vi "multiColorWormSaveSettings.vi"(1 "piezoPosition":dbl[](array[numeric]), 2 "moleculesSequence":string[](array[string])) -> ()   [LabVIEW 2017]
uses:
  globalUtilities.vi
  <vilib>/Utility/file.llb/Write Delimited Spreadsheet (DBL).vi
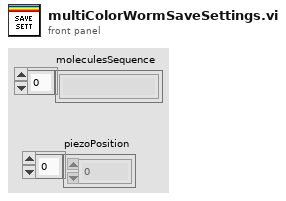
[diagram p1: front panel]
types:
  T1 = enum16{"open", "replace", "create", "open or create", "replace or create", "replace or create with confirmation"}
  T2 = cluster{"laserWavelength (nm)":dbl, "laserPower (mW)":dbl, "sliderPosition":u16}[]
  T3 = cluster{"laserWavelength":dbl, "exposureTime":dbl, "filterWheelPosition":u8, "name":string, "exposureTimeMultiplier":dbl}[]
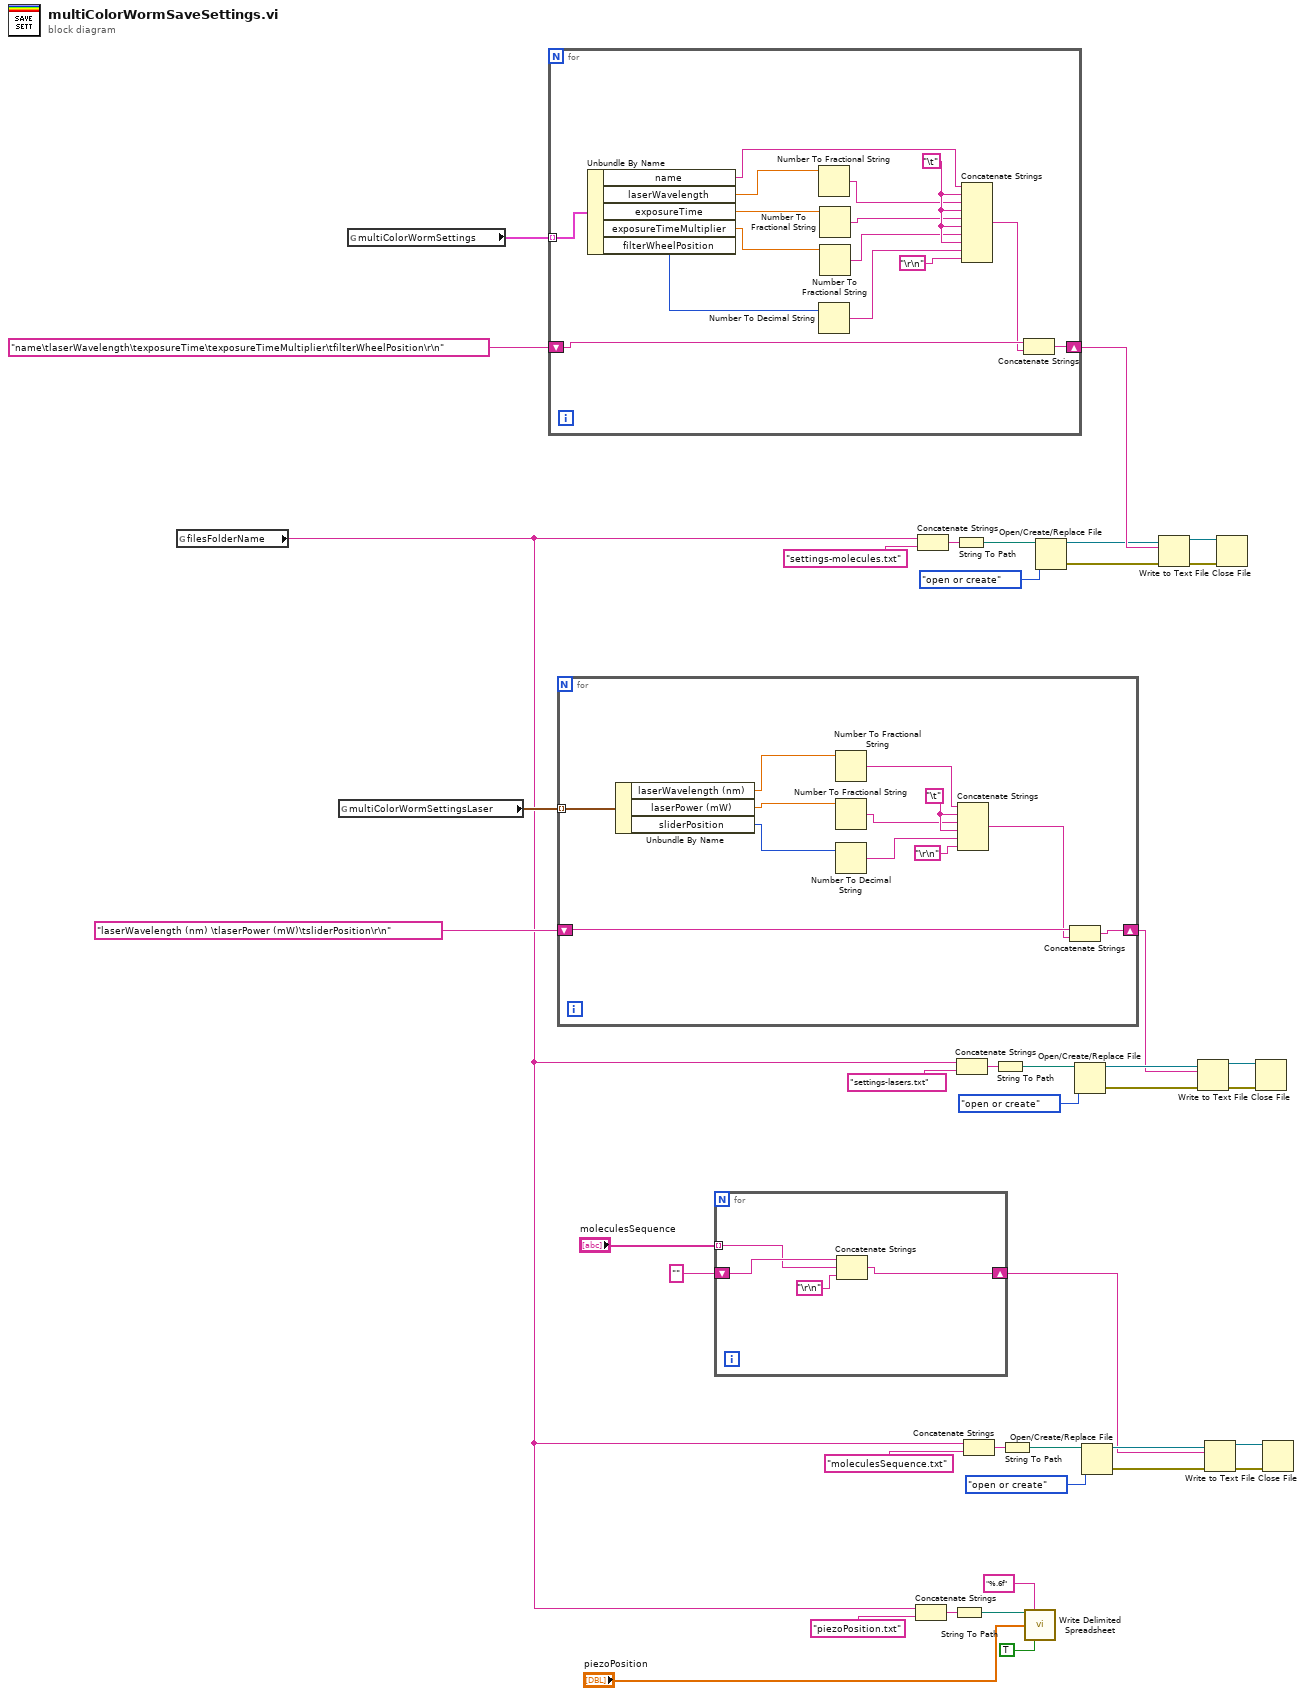
[diagram p0: block diagram]
diagram:
  n1 = global read "globalUtilities.vi" "filesFolderName"() -> (w5:string)
  n2 = global read "globalUtilities.vi" "multiColorWormSettingsLaser"() -> (w29:T2)
  n3 = global read "globalUtilities.vi" "multiColorWormSettings"() -> (w40:T3)
  n4 = for {
    tunnel: w40 -> [w55] mode=indexing
    shift-right: [w43] -> w38
    shift-left: "name\tlaserWavelength\texposureTime\texposureTimeMultiplier\tfilterWheelPosition\r\n" -> [w42]
    w49 = "\t"
    n5 = Unbundle By Name(w55) -> ("name"=w50:string, "laserWavelength"=w54:dbl, "exposureTime"=w53:dbl, "exposureTimeMultiplier"=w52:dbl, "filterWheelPosition"=w51:u8)
    n6 = Number To Fractional String(number=w54) -> (F-format string=w48:string)  [unwired: 3 in]
    n7 = Number To Decimal String(number=w51) -> (decimal integer string=w45:string)  [unwired: 1 in]
    n8 = Number To Fractional String(number=w53) -> (F-format string=w47:string)  [unwired: 3 in]
    n9 = Number To Fractional String(number=w52) -> (F-format string=w46:string)  [unwired: 3 in]
    n10 = Concatenate Strings(w50, w49, w48, w49, w47, w49, w46, w49, w45, "\r\n") -> (w41:string)
    n11 = Concatenate Strings(w42, w41) -> (w43:string)
  }
  n12 = for {
    tunnel: w29 -> [w67] mode=indexing
    shift-right: [w56] -> w19
    shift-left: "laserWavelength (nm) \tlaserPower (mW)\tsliderPosition\r\n" -> [w58]
    w63 = "\t"
    n13 = Unbundle By Name(w67) -> ("laserWavelength (nm)"=w66:dbl, "laserPower (mW)"=w65:dbl, "sliderPosition"=w64:u16)
    n14 = Number To Fractional String(number=w66) -> (F-format string=w62:string)  [unwired: 3 in]
    n15 = Number To Fractional String(number=w65) -> (F-format string=w61:string)  [unwired: 3 in]
    n16 = Number To Decimal String(number=w64) -> (decimal integer string=w60:string)  [unwired: 1 in]
    n17 = Concatenate Strings(w62, w63, w61, w63, w60, "\r\n") -> (w57:string)
    n18 = Concatenate Strings(w58, w57) -> (w56:string)
  }
  n19 = for {
    tunnel: "moleculesSequence" -> [w70] mode=indexing
    shift-right: [w68] -> w8
    shift-left: "" -> [w71]
    n20 = Concatenate Strings(w71, w70, "\r\n") -> (w68:string)
  }
  n21 = Concatenate Strings(w5, "piezoPosition.txt" ("string")) -> (w7:string)
  n22 = Concatenate Strings(w5, "settings-molecules.txt" ("string")) -> (w36:string)
  n23 = String To Path(string=w7) -> (path=w4:path)
  n24 = String To Path(string=w36) -> (path=w35:path)
  n25 = Concatenate Strings(w5, "settings-lasers.txt" ("string")) -> (w21:string)
  n26 = Concatenate Strings(w5, "moleculesSequence.txt" ("string")) -> (w15:string)
  n27 = String To Path(string=w21) -> (path=w22:path)
  n28 = String To Path(string=w15) -> (path=w14:path)
  n29 = call-poly <vilib>:"Write Delimited Spreadsheet.vi"("file path (dialog if empty)"=w4, "format (%.3f)"="%.6f", "1D data"="piezoPosition", "transpose? (no:F)"=TRUE) -> ()  [unwired: 10 in, 2 out]
  n30 = Open/Create/Replace File(file path (use dialog)=w35, operation (0:open)=T1."open or create") -> (refnum out=w33:refnum<file>, error out=w32:errorcluster)  [unwired: 4 in, 1 out]
  n31 = Open/Create/Replace File(file path (use dialog)=w22, operation (0:open)=T1."open or create") -> (refnum out=w24:refnum<file>, error out=w25:errorcluster)  [unwired: 4 in, 1 out]
  n32 = Open/Create/Replace File(file path (use dialog)=w14, operation (0:open)=T1."open or create") -> (refnum out=w12:refnum<file>, error out=w11:errorcluster)  [unwired: 4 in, 1 out]
  n33 = Write to Text File(file (use dialog)=w33, text=w38, error in=w32) -> (refnum out=w30:refnum<file>, error out=w31:errorcluster)  [unwired: 1 in, 1 out]
  n34 = Write to Text File(file (use dialog)=w24, text=w19, error in=w25) -> (refnum out=w27:refnum<file>, error out=w26:errorcluster)  [unwired: 1 in, 1 out]
  n35 = Write to Text File(file (use dialog)=w12, text=w8, error in=w11) -> (refnum out=w9:refnum<file>, error out=w10:errorcluster)  [unwired: 1 in, 1 out]
  n36 = Close File(refnum=w30, error in=w31) -> ()  [unwired: 2 out]
  n37 = Close File(refnum=w27, error in=w26) -> ()  [unwired: 2 out]
  n38 = Close File(refnum=w9, error in=w10) -> ()  [unwired: 2 out]
